vi "CommandList.vi"(0 "UR CB-Series In":refnum<class "UR CB-Series.lvclass">) -> (14 "UR CB-Series Out":refnum<class "UR CB-Series.lvclass">, 19 "Compatible Commands":T1[](array[typedef])=[{"Command"="Load", "Input"=FALSE, "Input Type"="", "Remote Mode Required"=FALSE, "Min Version"={"Major"=0, "Minor"=0, "Fix"=0, "Build"=0}, "Deprecated"=FALSE}, {"Command"="Play", "Input"=FALSE, "Input Type"="", "Remote Mode Required"=FALSE, "Min Version"={"Major"=0, "Minor"=0, "Fix"=0, "Build"=0}, "Deprecated"=FALSE}, {"Command"="Stop", "Input"=FALSE, "Input Type"="", "Remote Mode Required"=FALSE, "Min Version"={"Major"=0, "Minor"=0, "Fix"=0, "Build"=0}, "Deprecated"=FALSE}, {"Command"="Pause", "Input"=FALSE, "Input Type"="", "Remote Mode Required"=FALSE, "Min Version"={"Major"=0, "Minor"=0, "Fix"=0, "Build"=0}, "Deprecated"=FALSE}, {"Command"="Quit", "Input"=FALSE, "Input Type"="", "Remote Mode Required"=FALSE, "Min Version"={"Major"=0, "Minor"=0, "Fix"=0, "Build"=0}, "Deprecated"=FALSE}, {"Command"="Shutdown", "Input"=FALSE, "Input Type"="", "Remote Mode Required"=FALSE, "Min Version"={"Major"=0, "Minor"=0, "Fix"=0, "Build"=0}, "Deprecated"=FALSE}, {"Command"="Running", "Input"=FALSE, "Input Type"="", "Remote Mode Required"=FALSE, "Min Version"={"Major"=0, "Minor"=0, "Fix"=0, "Build"=0}, "Deprecated"=FALSE}, {"Command"="Robotmode", "Input"=FALSE, "Input Type"="", "Remote Mode Required"=FALSE, "Min Version"={"Major"=0, "Minor"=0, "Fix"=0, "Build"=0}, "Deprecated"=FALSE}, {"Command"="get loaded program", "Input"=FALSE, "Input Type"="", "Remote Mode Required"=FALSE, "Min Version"={"Major"=0, "Minor"=0, "Fix"=0, "Build"=0}, "Deprecated"=FALSE}, {"Command"="popup", "Input"=TRUE, "Input Type"="<popup-text>", "Remote Mode Required"=FALSE, "Min Version"={"Major"=0, "Minor"=0, "Fix"=0, "Build"=0}, "Deprecated"=FALSE}, {"Command"="close popup", "Input"=FALSE, "Input Type"="", "Remote Mode Required"=FALSE, "Min Version"={"Major"=0, "Minor"=0, "Fix"=0, "Build"=0}, "Deprecated"=FALSE}, {"Command"="addToLog", "Input"=FALSE, "Input Type"="<log-message>", "Remote Mode Required"=FALSE, "Min Version"={"Major"=0, "Minor"=0, "Fix"=0, "Build"=0}, "Deprecated"=FALSE}, {"Command"="IsProgramSaved", "Input"=FALSE, "Input Type"="", "Remote Mode Required"=FALSE, "Min Version"={"Major"=0, "Minor"=0, "Fix"=0, "Build"=0}, "Deprecated"=FALSE}, {"Command"="programState", "Input"=FALSE, "Input Type"="", "Remote Mode Required"=FALSE, "Min Version"={"Major"=0, "Minor"=0, "Fix"=0, "Build"=0}, "Deprecated"=FALSE}, {"Command"="PolyscopeVersion", "Input"=FALSE, "Input Type"="", "Remote Mode Required"=FALSE, "Min Version"={"Major"=0, "Minor"=0, "Fix"=0, "Build"=0}, "Deprecated"=FALSE}, {"Command"="set operational mode", "Input"=FALSE, "Input Type"="<mode>", "Remote Mode Required"=FALSE, "Min Version"={"Major"=0, "Minor"=0, "Fix"=0, "Build"=0}, "Deprecated"=FALSE}, {"Command"="clear operational mode", "Input"=FALSE, "Input Type"="", "Remote Mode Required"=FALSE, "Min Version"={"Major"=0, "Minor"=0, "Fix"=0, "Build"=0}, "Deprecated"=FALSE}, {"Command"="power on", "Input"=FALSE, "Input Type"="", "Remote Mode Required"=FALSE, "Min Version"={"Major"=0, "Minor"=0, "Fix"=0, "Build"=0}, "Deprecated"=FALSE}, {"Command"="power off", "Input"=FALSE, "Input Type"="", "Remote Mode Required"=FALSE, "Min Version"={"Major"=0, "Minor"=0, "Fix"=0, "Build"=0}, "Deprecated"=FALSE}])   [LabVIEW 2019, in "UR CB-Series.lvclass"]
uses:
  UR CB-Series.lvclass
  Universal Robot/PolyScopeCommand.ctl
  Universal Robot/PolyScopeVersion.ctl
  Universal Robot/Universal Robot.lvclass
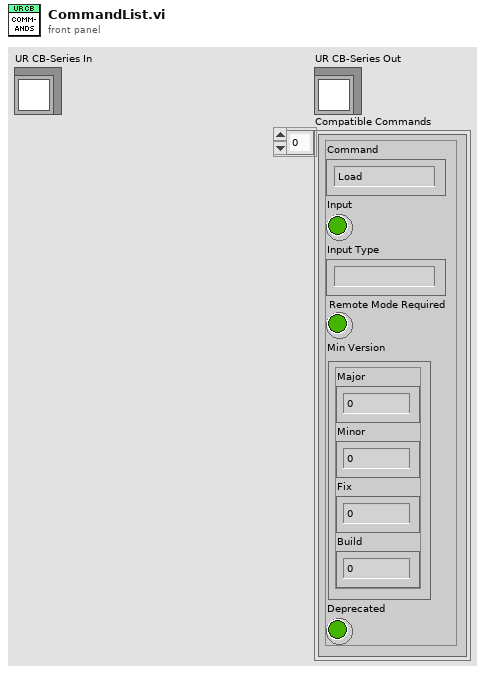
[diagram p1: front panel]
types:
  T1 = typedef "Universal Robot.lvclass/PolyScopeCommand.ctl" = cluster{"Command":string, "Input":bool, "Input Type":string, "Remote Mode Required":bool, "Min Version":T2, "Deprecated":bool}
  T2 = typedef "Universal Robot.lvclass/PolyScopeVersion.ctl" = cluster{"Major":i32, "Minor":i32, "Fix":i32, "Build":i32}
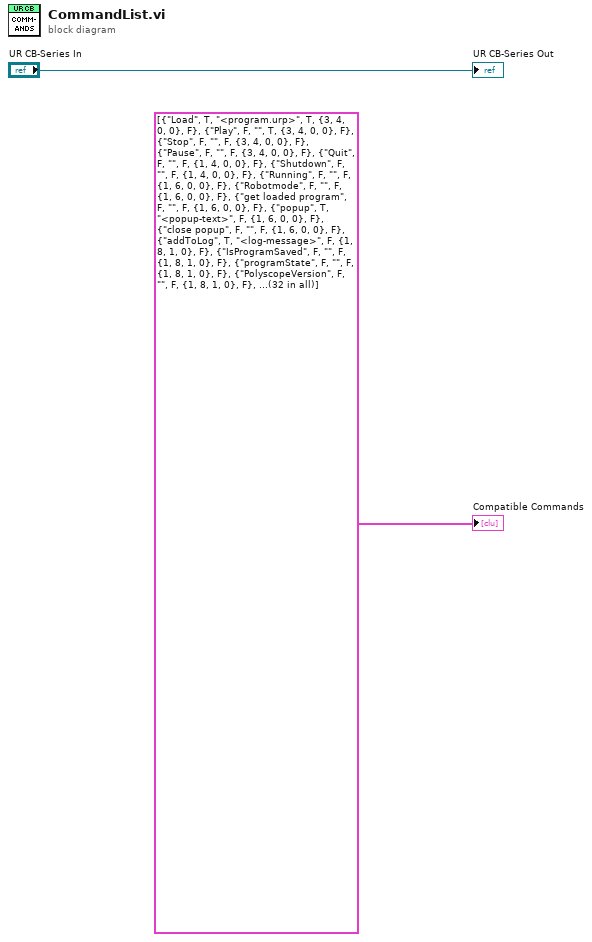
[diagram p0: block diagram]
diagram:
  "Compatible Commands" <- T1[] [{"Command"="Load", "Input"=TRUE, "Input Type"="<program.urp>", "Remote Mode Required"=TRUE, "Min Version"={"Major"=3, "Minor"=4, "Fix"=0, "Build"=0}, "Deprecated"=FALSE}, {"Command"="Play", "Input"=FALSE, "Input Type"="", "Remote Mode Required"=TRUE, "Min Version"={"Major"=3, "Minor"=4, "Fix"=0, "Build"=0}, "Deprecated"=FALSE}, {"Command"="Stop", "Input"=FALSE, "Input Type"="", "Remote Mode Required"=FALSE, "Min Version"={"Major"=3, "Minor"=4, "Fix"=0, "Build"=0}, "Deprecated"=FALSE}, {"Command"="Pause", "Input"=FALSE, "Input Type"="", "Remote Mode Required"=FALSE, "Min Version"={"Major"=3, "Minor"=4, "Fix"=0, "Build"=0}, "Deprecated"=FALSE}, {"Command"="Quit", "Input"=FALSE, "Input Type"="", "Remote Mode Required"=FALSE, "Min Version"={"Major"=1, "Minor"=4, "Fix"=0, "Build"=0}, "Deprecated"=FALSE}, {"Command"="Shutdown", "Input"=FALSE, "Input Type"="", "Remote Mode Required"=FALSE, "Min Version"={"Major"=1, "Minor"=4, "Fix"=0, "Build"=0}, "Deprecated"=FALSE}, {"Command"="Running", "Input"=FALSE, "Input Type"="", "Remote Mode Required"=FALSE, "Min Version"={"Major"=1, "Minor"=6, "Fix"=0, "Build"=0}, "Deprecated"=FALSE}, {"Command"="Robotmode", "Input"=FALSE, "Input Type"="", "Remote Mode Required"=FALSE, "Min Version"={"Major"=1, "Minor"=6, "Fix"=0, "Build"=0}, "Deprecated"=FALSE}, {"Command"="get loaded program", "Input"=FALSE, "Input Type"="", "Remote Mode Required"=FALSE, "Min Version"={"Major"=1, "Minor"=6, "Fix"=0, "Build"=0}, "Deprecated"=FALSE}, {"Command"="popup", "Input"=TRUE, "Input Type"="<popup-text>", "Remote Mode Required"=FALSE, "Min Version"={"Major"=1, "Minor"=6, "Fix"=0, "Build"=0}, "Deprecated"=FALSE}, {"Command"="close popup", "Input"=FALSE, "Input Type"="", "Remote Mode Required"=FALSE, "Min Version"={"Major"=1, "Minor"=6, "Fix"=0, "Build"=0}, "Deprecated"=FALSE}, {"Command"="addToLog", "Input"=TRUE, "Input Type"="<log-message>", "Remote Mode Required"=FALSE, "Min Version"={"Major"=1, "Minor"=8, "Fix"=1, "Build"=0}, "Deprecated"=FALSE}, {"Command"="IsProgramSaved", "Input"=FALSE, "Input Type"="", "Remote Mode Required"=FALSE, "Min Version"={"Major"=1, "Minor"=8, "Fix"=1, "Build"=0}, "Deprecated"=FALSE}, {"Command"="programState", "Input"=FALSE, "Input Type"="", "Remote Mode Required"=FALSE, "Min Version"={"Major"=1, "Minor"=8, "Fix"=1, "Build"=0}, "Deprecated"=FALSE}, {"Command"="PolyscopeVersion", "Input"=FALSE, "Input Type"="", "Remote Mode Required"=FALSE, "Min Version"={"Major"=1, "Minor"=8, "Fix"=1, "Build"=0}, "Deprecated"=FALSE}, {"Command"="set operational mode", "Input"=TRUE, "Input Type"="<mode>", "Remote Mode Required"=FALSE, "Min Version"={"Major"=5, "Minor"=0, "Fix"=0, "Build"=0}, "Deprecated"=FALSE}, {"Command"="clear operational mode", "Input"=FALSE, "Input Type"="", "Remote Mode Required"=FALSE, "Min Version"={"Major"=5, "Minor"=0, "Fix"=0, "Build"=0}, "Deprecated"=FALSE}, {"Command"="power on", "Input"=FALSE, "Input Type"="", "Remote Mode Required"=TRUE, "Min Version"={"Major"=5, "Minor"=0, "Fix"=0, "Build"=0}, "Deprecated"=FALSE}, {"Command"="power off", "Input"=FALSE, "Input Type"="", "Remote Mode Required"=FALSE, "Min Version"={"Major"=5, "Minor"=0, "Fix"=0, "Build"=0}, "Deprecated"=FALSE}, {"Command"="brake release", "Input"=TRUE, "Input Type"="", "Remote Mode Required"=FALSE, "Min Version"={"Major"=5, "Minor"=0, "Fix"=0, "Build"=0}, "Deprecated"=FALSE}, {"Command"="safetymode", "Input"=FALSE, "Input Type"="", "Remote Mode Required"=FALSE, "Min Version"={"Major"=5, "Minor"=0, "Fix"=0, "Build"=0}, "Deprecated"=TRUE}, {"Command"="safetystatus", "Input"=FALSE, "Input Type"="", "Remote Mode Required"=FALSE, "Min Version"={"Major"=5, "Minor"=4, "Fix"=0, "Build"=0}, "Deprecated"=FALSE}, {"Command"="unlock protective stop", "Input"=FALSE, "Input Type"="", "Remote Mode Required"=FALSE, "Min Version"={"Major"=5, "Minor"=0, "Fix"=0, "Build"=0}, "Deprecated"=FALSE}, {"Command"="close safety popup", "Input"=FALSE, "Input Type"="", "Remote Mode Required"=FALSE, "Min Version"={"Major"=5, "Minor"=0, "Fix"=0, "Build"=0}, "Deprecated"=FALSE}, {"Command"="load installation", "Input"=TRUE, "Input Type"="<default.installation>", "Remote Mode Required"=TRUE, "Min Version"={"Major"=5, "Minor"=0, "Fix"=0, "Build"=0}, "Deprecated"=FALSE}, {"Command"="restart safety", "Input"=FALSE, "Input Type"="", "Remote Mode Required"=FALSE, "Min Version"={"Major"=5, "Minor"=1, "Fix"=0, "Build"=0}, "Deprecated"=FALSE}, {"Command"="get operational mode", "Input"=FALSE, "Input Type"="", "Remote Mode Required"=TRUE, "Min Version"={"Major"=5, "Minor"=6, "Fix"=0, "Build"=0}, "Deprecated"=FALSE}, {"Command"="is in remote control", "Input"=FALSE, "Input Type"="", "Remote Mode Required"=FALSE, "Min Version"={"Major"=5, "Minor"=6, "Fix"=0, "Build"=0}, "Deprecated"=FALSE}, {"Command"="get serial number", "Input"=FALSE, "Input Type"="", "Remote Mode Required"=FALSE, "Min Version"={"Major"=5, "Minor"=6, "Fix"=0, "Build"=0}, "Deprecated"=FALSE}, {"Command"="get robot model", "Input"=FALSE, "Input Type"="", "Remote Mode Required"=FALSE, "Min Version"={"Major"=5, "Minor"=6, "Fix"=0, "Build"=0}, "Deprecated"=FALSE}, {"Command"="generate flight report", "Input"=TRUE, "Input Type"="<report type>", "Remote Mode Required"=FALSE, "Min Version"={"Major"=5, "Minor"=8, "Fix"=0, "Build"=0}, "Deprecated"=FALSE}, {"Command"="generate support file", "Input"=TRUE, "Input Type"="<directory path>", "Remote Mode Required"=FALSE, "Min Version"={"Major"=5, "Minor"=8, "Fix"=0, "Build"=0}, "Deprecated"=FALSE}]
  "UR CB-Series Out" <- "UR CB-Series In"
